vi "Main.vi"() -> ()   [LabVIEW 2024]
doc: "Program analizuje plik z danymi z treningu przetwarza je, uporządkowuje w tablicach i tworzy na jego podstawie wykresy. Może również zapisać tabelę lub wykres, a także wyświetlić historię treningów."
uses:
  zad_3-labview/klaster 4.ctl
  zad_3-labview/klaster.ctl
  zad_3-labview/klaster 2.ctl
  Documents/LabVIEW Data/HR Monitor/controls/VN State.ctl
  <vilib>/Utility/file.llb/Write Delimited Spreadsheet (string).vi
panel:
  in  "Show history":bool
  in  "error in (no error)":errorcluster
  in  "HR Data Structure":T1={"Runer's Data"={"Name"="", "Age"=0}, "HR Max"=0, "Raw Data"={"Time"=[], "Bpm"=[]}, "% HR MAX "=[], "HR Zones "=[], "no of points"=[], "Heart Rate Zone No 2"=[1, 2, 3, 4, 5], "History"=[["training number", "HR Max value", "HR Mean value"], ["", "", ""]], "number history"=0}
  in  "Save Results":bool
  in  "New Traning":bool
  in  "Stop":bool
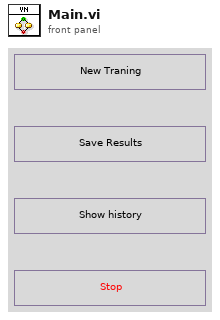
[diagram p1: front panel]
types:
  T1 = typedef "klaster 4.ctl" = cluster{"Runer's Data":T2, "HR Max":i32, "Raw Data":T3, "% HR MAX ":dbl[], "HR Zones ":string[][], "no of points":dbl[], "Heart Rate Zone No 2":i32[], "History":string[][], "number history":i32}
  T2 = typedef "klaster.ctl" = cluster{"Name":string, "Age":i32}
  T3 = typedef "klaster 2.ctl" = cluster{"Time":timestamp[], "Bpm":i32[]}
  T4 = typedef "VN State.ctl" = enum16{"Aplication Error", "Initialize", "Idle", "Analize New Traning", "Show history", "Save", "Error Handling", "Stop"}
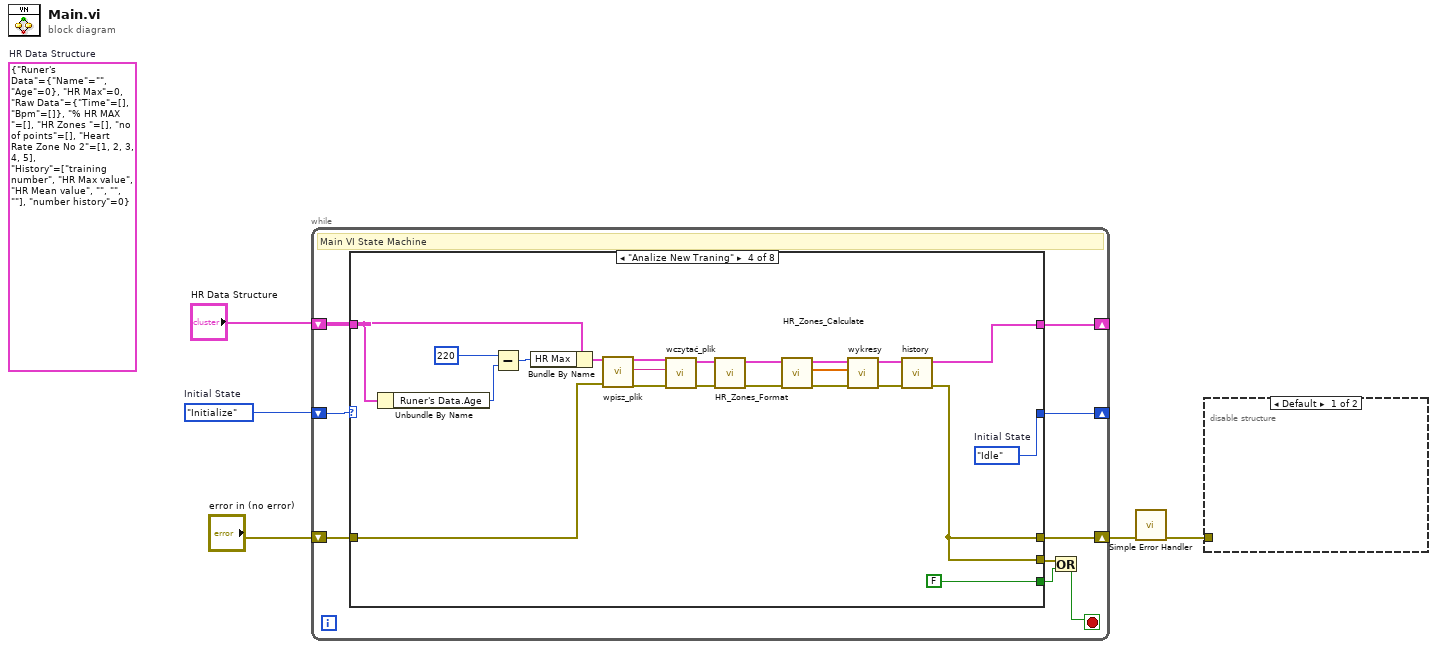
[diagram p0: block diagram]
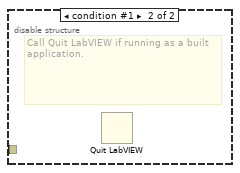
[diagram p2: hidden frame]
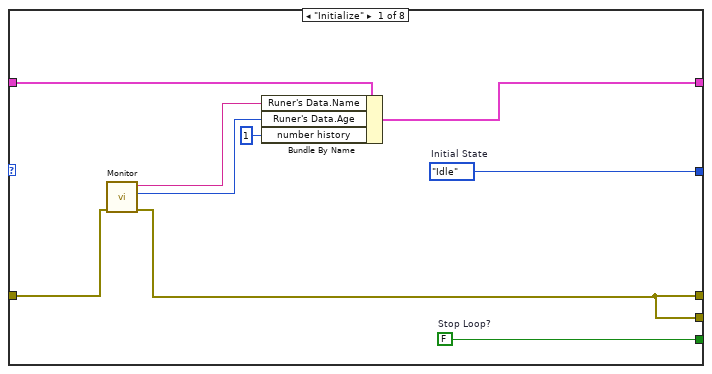
[diagram p3: hidden frame]
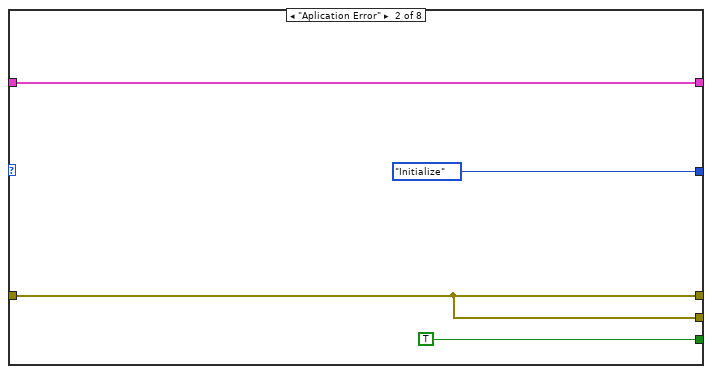
[diagram p4: hidden frame]
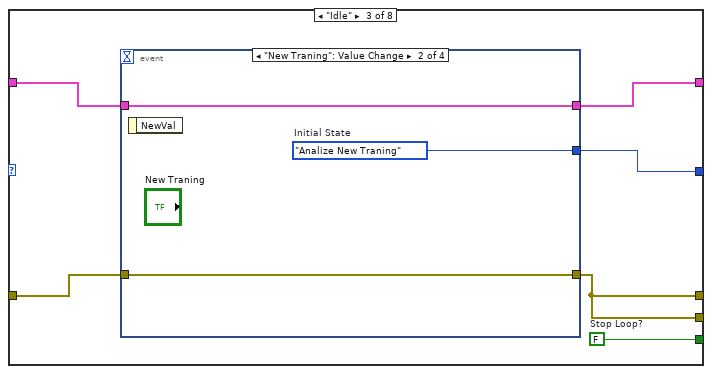
[diagram p5: hidden frame]
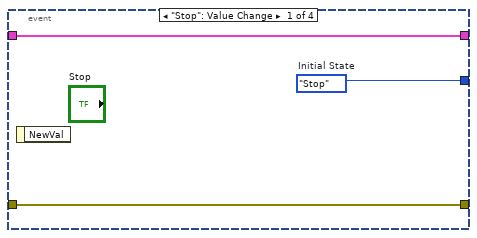
[diagram p6: hidden frame]
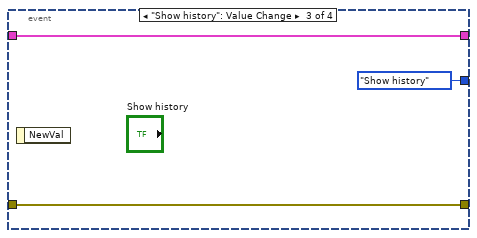
[diagram p7: hidden frame]
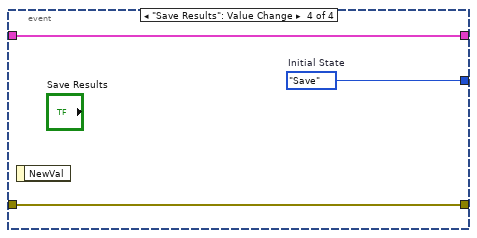
[diagram p8: hidden frame]
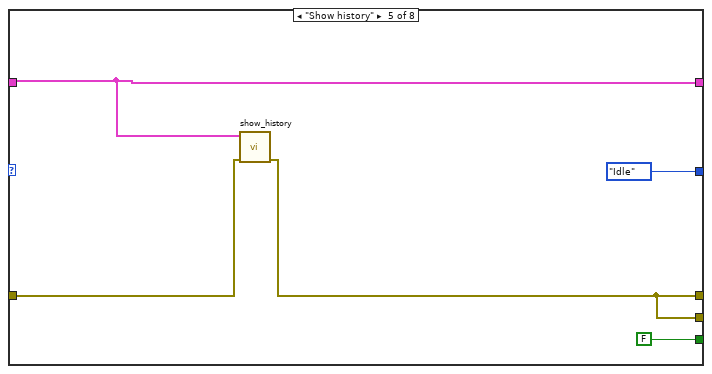
[diagram p9: hidden frame]
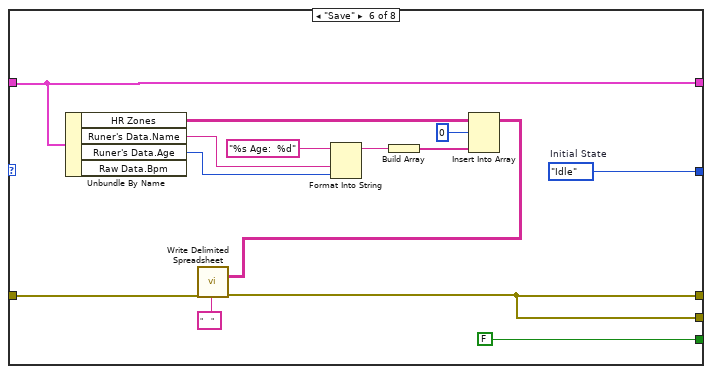
[diagram p10: hidden frame]
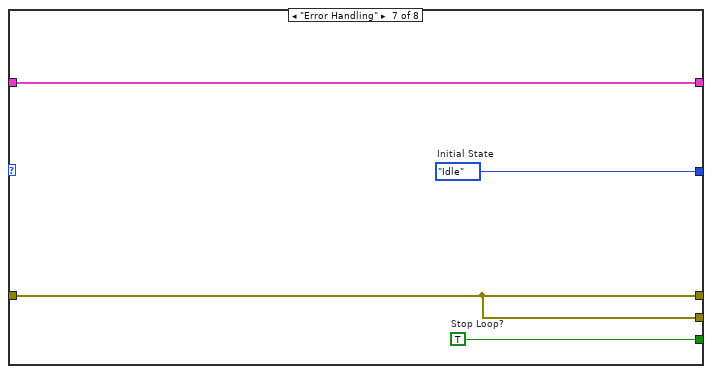
[diagram p11: hidden frame]
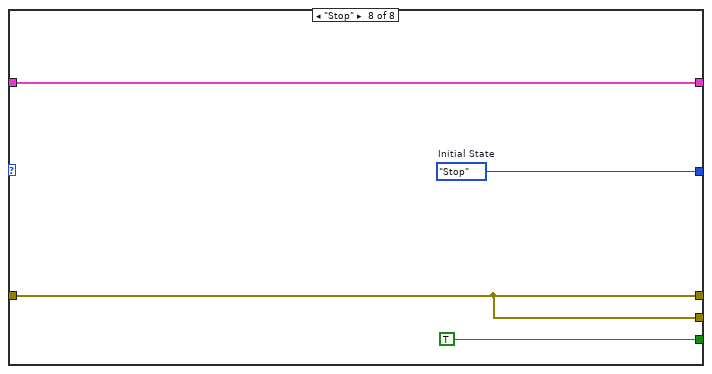
[diagram p12: hidden frame]
diagram:
  (unwired) T1 {"Runer's Data"={"Name"="", "Age"=0}, "HR Max"=0, "Raw Data"={"Time"=[], "Bpm"=[]}, "% HR MAX "=[], "HR Zones "=[], "no of points"=[], "Heart Rate Zone No 2"=[1, 2, 3, 4, 5], "History"=[["training number", "HR Max value", "HR Mean value"], ["", "", ""]], "number history"=0}  # HR Data Structure
  w5 = VN_State."Initialize"  # Initial State
  n1 = while {
    shift-right: [w7] -> _
    shift-left: w5 -> [w14]
    shift-right: [w12] -> _
    shift-left: "HR Data Structure" -> [w13]
    shift-right: [w8] -> w1
    shift-left: "error in (no error)" -> [w11]
    stop <- w9 stop-if-true
    # "Main VI State Machine"
    n2 = case shown="\"Analize New Traning\"" w14 {
      tunnel: [w23 TRUE ("Stop Loop?") w33 FALSE ("Stop Loop?") FALSE ("Stop Loop?") FALSE ("Stop Loop?") w89 TRUE] -> w10
      tunnel: w13 -> [w18 w27 w32 w58 w70 w81 w90 w94]
      tunnel: [w21 w27 w31 w48 w70 w81 w90 w94] -> w12
      tunnel: w11 -> [w20 w26 w30 w56 w69 w83 w87 w91]
      tunnel: [w19 w26 w28 w47 w68 w82 w87 w91] -> w8
      tunnel: [w22 VN_State."Initialize" ("Initial State") w29 w66 VN_State."Idle" ("Initial State") w85 w88 w93] -> w7
      tunnel: [w19 w26 w28 w47 w68 w82 w87 w91] -> w6
      frame "Initialize" {
        w22 = VN_State."Idle"  # Initial State
        w23 = FALSE  # Stop Loop?
        # "Initialize - Initialize the application."
        n3 = call "Monitor.vi"("error In"=w20) -> ("error Out"=w19:errorcluster, "Wiek 2"=w16:i32, "imie 2"=w17:string)  [unwired: 8 in]
        n4 = Bundle By Name(cluster=w18, "Runer's Data.Name"=w17, "Runer's Data.Age"=w16, "number history"=1) -> (w21:T1)
      }
      frame "Aplication Error" {
      }
      frame "Idle" {
        w33 = FALSE  # Stop Loop?
        # "Wait for Event - Use an Event Structure to monitor the user interface for events that run different states of the state machine."
        n5 = event shown="[1] \"New Traning\": Value Change" {
          selector: _ -> [_ _ _ _]
          dyn-events: _ -> [_ _ _ _]
          timeout: _ -> [_ _ _ _]
          tunnel: w32 -> [w36 w37 w40 w43]
          tunnel: [w36 w37 w40 w43] -> w31
          tunnel: w30 -> [w35 w38 w42 w45]
          tunnel: [w35 w38 w42 w45] -> w28
          tunnel: [w34 w39 VN_State."Show history" ("Initial State") w44] -> w29
          event "Stop": Value Change {
            w34 = VN_State."Stop"  # Initial State
            n6 = event-data() -> ()  [unwired: 1 in, 1 out]
          }
          event "New Traning": Value Change {
            w39 = VN_State."Analize New Traning"  # Initial State
            n7 = event-data() -> ()  [unwired: 1 in, 1 out]
          }
          event "Show history": Value Change {
            n8 = event-data() -> ()  [unwired: 1 in, 1 out]
          }
          event "Save Results": Value Change {
            w44 = VN_State."Save"  # Initial State
            n9 = event-data() -> ()  [unwired: 1 in, 1 out]
          }
        }
      }
      frame "Analize New Traning" {
        w66 = VN_State."Idle"  # Initial State
        # "User State 1 - Replace this state with functionality for your own application."
        n10 = Unbundle By Name(w58) -> ("Runer's Data.Age"=w60:i32)
        n11 = Subtract(x=220, y=w60) -> (x-y=w59:i32)
        n12 = Bundle By Name(cluster=w58, "HR Max"=w59) -> (w55:T1)
        n13 = call "wpisz_plik.vi"("error in"=w56, "HR Data Structure"=w55) -> ("error out"=w57:errorcluster, "text"=w53:string, "HR Data Structure 2"=w54:T1)  [unwired: 7 in]
        n14 = call "wczytać_plik.vi"("error in"=w57, "String"=w53, "wejście cluster"=w54) -> ("error  out"=w63:errorcluster, "wyjście cluster"=w64:T1)  [unwired: 7 in]
        n15 = call "HR_Zones_Format.vi"("error in (no error)"=w63, "wejście"=w64) -> ("error out"=w61:errorcluster, "wyjście"=w62:T1)  [unwired: 8 in]
        n16 = call "HR_Zones_Calculate.vi"("error in (no error)"=w61, "wejście"=w62) -> ("error out"=w51:errorcluster, "x*y"=w46:dbl[], "wyjście"=w52:T1)  [unwired: 7 in]
        n17 = call "wykresy.vi"("error in (no error)"=w51, "x*y"=w46, "wyjście"=w52) -> ("error in (no error) 2"=w49:errorcluster, "wyjście 2"=w50:T1)  [unwired: 7 in]
        n18 = call "history.vi"("error in (no error)"=w49, "HR Data Structure"=w50) -> ("error in (no error) 2"=w47:errorcluster, "output cluster"=w48:T1)  [unwired: 8 in]
      }
      frame "Show history" {
        n19 = call "show_history.vi"("error in (no error)"=w69, "HR Data Structure"=w70) -> ("error in (no error) 2"=w68:errorcluster)  [unwired: 9 in]
      }
      frame "Save" {
        w85 = VN_State."Idle"  # Initial State
        # "User State 2 - Replace this state with functionality for your own application."
        n20 = Unbundle By Name(w81) -> ("HR Zones"=w80:string[][], "Runer's Data.Name"=w75:string, "Runer's Data.Age"=w73:i32)  [unwired: 1 out]
        n21 = Format Into String(format string="%s Age:  %d", w75, w73) -> (resulting string=w76:string)  [unwired: 2 in, 1 out]
        n22 = Build Array(w76) -> (w77:string[])
        n23 = Insert Into Array(array=w80, index (row)=0 ("index (col)"), new element=w77) -> (w79:string[][])  [unwired: 1 in]
        n24 = call-poly <vilib>:"Write Delimited Spreadsheet.vi"("2D data"=w79, "error in (no error)"=w83, "delimiter (\\t)"="    " ("delimiter (\\t)")) -> ("error out"=w82:errorcluster)  [unwired: 11 in, 1 out]
      }
      frame "Error Handling" {
        w88 = VN_State."Idle"  # Initial State
        w89 = TRUE  # Stop Loop?
        # "Exit - Exit the application."
      }
      frame "Stop" {
        w93 = VN_State."Stop"  # Initial State
      }
    }
    n25 = Or(x=w6, y=w10) -> (x .or. y?=w9:bool)
  }
  n26 = call <vilib>:"Simple Error Handler.vi"("error in (no error)"=w1) -> ("error out"=w4:errorcluster)  [unwired: 4 in, 4 out]
  n27 = disable-structure shown="Default" {
    disable-tunnel: w4 -> [_ _]
    frame condition #0 (active) {
    }
    frame condition #1 {
      # "Call Quit LabVIEW if running as a built application."
      n28 = Quit LabVIEW() -> ()  [unwired: 1 in]
    }
  }
